vi "OutlineInComments.vi"   [LabVIEW 2010]
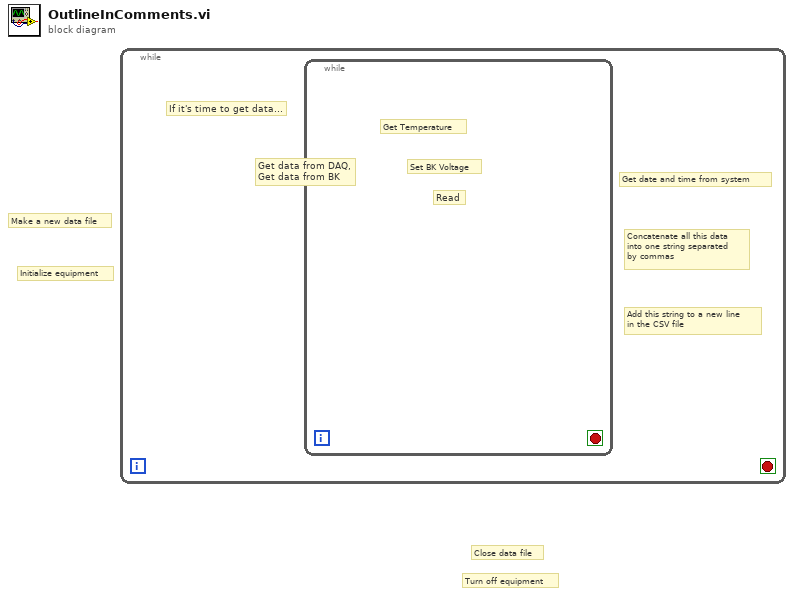
[diagram p0: block diagram]
diagram:
  # "Turn off equipment"
  # "Initialize equipment"
  # "Close data file"
  # "Make a new data file"
  n1 = while {
    stop <- _ stop-if-true
    # "Add this string to a new line\nin the CSV file"
    # "Concatenate all this data\ninto one string separated\nby commas"
    # "Get date and time from system"
    # "Get data from DAQ,\nGet data from BK"
    # "If it's time to get data..."
    n2 = while {
      stop <- _ stop-if-true
      # "Read"
      # "Set BK Voltage"
      # "Get Temperature"
    }
  }
